vi "Phasor Compute 1-Exp Array.vi"(8 "Error In":errorcluster, 9 "Gate & Decay Parameters":T1 {"A" format="%#_4g"; "s" format="%#_4g"; "sF" format="%#_4g"; "sR" format="%#_4g"; "t_i" format="%#_4g"; "t_0" format="%#_4g"; "tau" format="%#_4g"; "T" format="%#_4g"; "W" format="%#_4g"}, 11 "X":dbl[](array[numeric])) -> (0 "Error Out":errorcluster, 1 "A":dbl, 3 "1-Exp Array":dbl[](array[numeric]))   [LabVIEW 2021, in "Phasor.lvlib"]
uses:
  Phasor.lvlib
  Phasor Gate & Decay Parameters.ctl
  Phasor Gate Type.ctl
  Phasor IRF Model.ctl
  Graphs/XY Graph/XY Plot Data.ctl
  fcae3ab5-1fbf-4800-815c-dafd3fbe87f6.vi
  177a4ce5-ee60-417e-8343-56d2beb784de.vi
  fcae3ab5-1fbf-4800-815c-dafd3fbe87f6.vi/50f0d027-e7bb-44ec-924d-0efee2062fcf.vi
  Graphs/XY Graph/XY Graph Add-Ons.lvlib
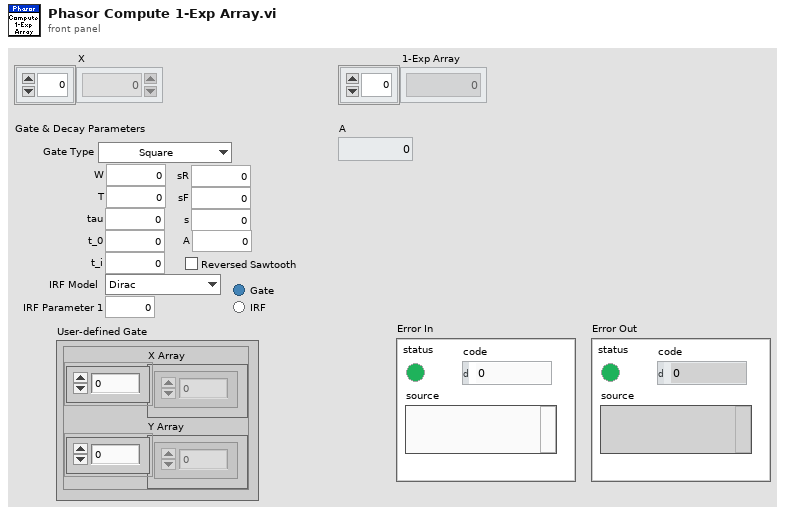
[diagram p1: front panel]
types:
  T1 = typedef "Phasor.lvlib/Phasor Gate & Decay Parameters.ctl" = cluster{"W":dbl, "T":dbl, "tau":dbl, "t_0":dbl, "Gate Type":T2, "t_i":dbl, "sR":dbl, "sF":dbl, "s":dbl, "Reversed Sawtooth":bool, "IRF Model":T3, "IRF Parameter 1":dbl, "User-defined Gate":T4, "Type of User-defined Function":enum32{"Gate", "IRF"}, "A":dbl}
  T2 = typedef "Phasor.lvlib/Phasor Gate Type.ctl" = enum16{"Square", "Finite Edge Square", "Finite Edge, Tilted Top Square", "Triangle", "Sawtooth", "User-defined"}
  T3 = typedef "Phasor.lvlib/Phasor IRF Model.ctl" = enum16{"Dirac", "Exponential"}
  T4 = typedef "XY Graph Add-Ons.lvlib/XY Plot Data.ctl" = cluster{"X Array":dbl[], "Y Array":dbl[]}
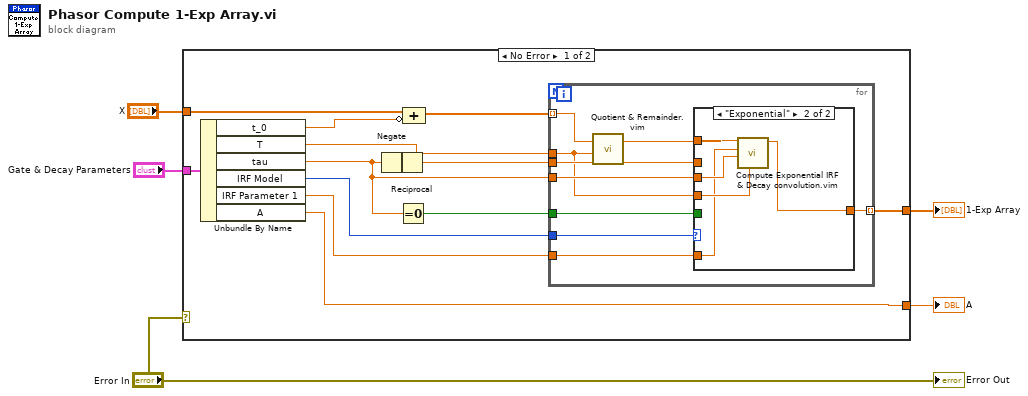
[diagram p0: block diagram]
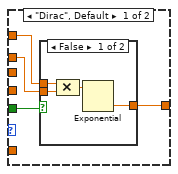
[diagram p2: hidden frame]
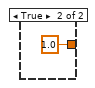
[diagram p3: hidden frame]
diagram:
  n1 = case shown="No Error" "Error In" {
    tunnel: "Gate & Decay Parameters" -> [w18 _]
    tunnel: "X" -> [w17 _]
    tunnel: [w15 _] -> w3
    tunnel: [w14 _] -> w2
    frame No Error {
      n2 = Unbundle By Name(w18) -> ("t_0"=w6:dbl, "T"=w16:dbl, "tau"=w12:dbl, "IRF Model"=w10:T3, "IRF Parameter 1"=w11:dbl, "A"=w15:dbl)
      n3 = Negate(x=w12) -> (-x=w8:dbl)
      n4 = Reciprocal(x=w8) -> (1/x=w9:dbl)
      n5 = Equal To 0?(x=w12) -> (x = 0?=w13:bool)
      n6 = Compound Arithmetic op=ADD(w17, invert w6) -> (w7:dbl[])
      n7 = for {
        tunnel: w16 -> [w19]
        tunnel: w9 -> [w22]
        tunnel: w7 -> [w20] mode=indexing
        tunnel: [w27] -> w14 mode=indexing
        tunnel: w10 -> [w26]
        tunnel: w11 -> [w25]
        tunnel: w12 -> [w24]
        tunnel: w13 -> [w21]
        n8 = call "Quotient & Remainder.vim"("y"=w19, "x"=w20) -> ("x - E(x/y)y"=w23:dbl)  [unwired: 1 out]
        n9 = case shown="\"Exponential\"" w26 {
          tunnel: [w30 w40] -> w27
          tunnel: w23 -> [w29 w41]
          tunnel: w25 -> [_ w37]
          tunnel: w24 -> [_ w39]
          tunnel: w19 -> [_ w38]
          tunnel: w22 -> [w31 _]
          tunnel: w21 -> [w28 _]
          frame "Dirac", Default {
            n10 = case shown="False" w28 {
              tunnel: w31 -> [w35 _]
              tunnel: [w34 1.0] -> w30
              tunnel: w29 -> [w33 _]
              frame False {
                n11 = Compound Arithmetic op=MULTIPLY(w33, w35) -> (w32:dbl)
                n12 = Exponential(1:w32) -> (0:w34:dbl)
              }
              frame True {
              }
            }
          }
          frame "Exponential" {
            n13 = call "Compute Exponential IRF & Decay convolution.vim"("Period: T"=w38, "lifetime: tau"=w39, "IRF time constant"=w37, "t"=w41) -> ("y(t)"=w40:dbl)  [unwired: 6 in, 1 out]
          }
        }
      }
    }
    frame Error {
    }
  }
  "A" <- w3
  "1-Exp Array" <- w2
  "Error Out" <- "Error In"
